vi "drive at angle.vi"() -> ()   [LabVIEW 2016]
uses:
  <vilib>/Rock Robotics/WPI/RobotDrive/WPI_RobotDriveDevRef.ctl
  <vilib>/Rock Robotics/WPI/MotorControl/WPI_MotorControlDeviceRef.ctl
  <vilib>/Rock Robotics/WPI/MotorControl/WPI_MotorControlType.ctl
  <vilib>/Rock Robotics/SystemInterfaces/DIO/FPGA_DIOPWMChannel.ctl
  <vilib>/Rock Robotics/WPI/PWM/WPI_PWMDeadband.ctl
  Robot Global Data.vi
  <vilib>/Rock Robotics/WPI/RobotDrive/WPI_RobotDriveArcadeDrive_Standard(NoSaturation).vi
panel:
  in  "angle":dbl
  in  "power(neg)":dbl
  in  "x inches":dbl
  in  "error in (no error)":errorcluster
  in  "RobotDriveDevRef":T1={"DevStatus"={"status"=FALSE, "code"=0, "source"=""}, "Motors[]"=[], "Square Inputs"=FALSE, "Max Output"=1.0}
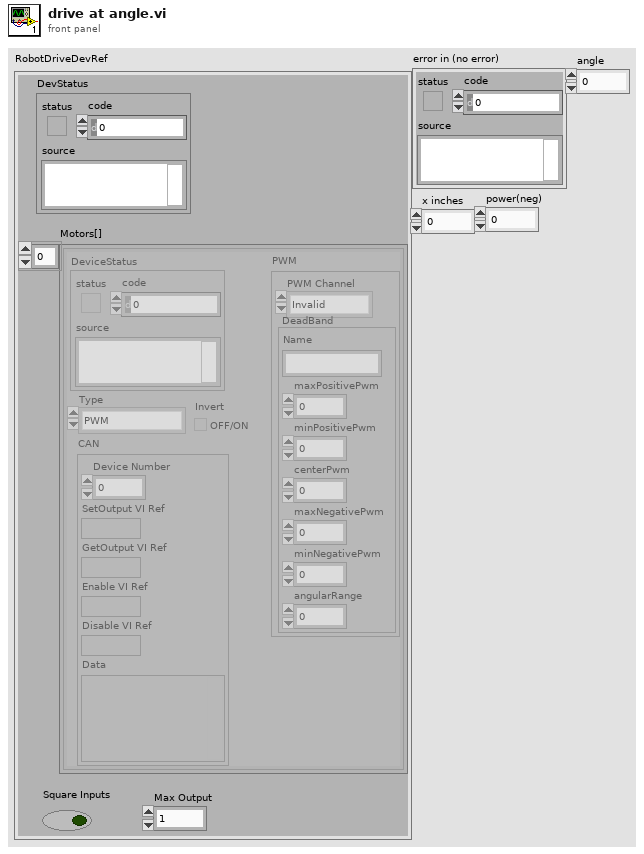
[diagram p1: front panel]
types:
  T1 = typedef "WPI_RobotDriveDevRef.ctl" = cluster{"DevStatus":errorcluster, "Motors[]":T2[], "Square Inputs":bool, "Max Output":dbl}
  T2 = typedef "WPI_MotorControlDeviceRef.ctl" = cluster{"DeviceStatus":errorcluster, "Type":T3, "PWM":cluster{"PWM Channel":T4, "DeadBand":T5}, "CAN":cluster{"Device Number":u8, "SetOutput VI Ref":variant, "GetOutput VI Ref":variant, "Enable VI Ref":variant, "Disable VI Ref":variant, "Data":variant}, "Invert":bool}
  T3 = typedef "WPI_MotorControlType.ctl" = enum16{"PWM", "CAN"}
  T4 = typedef "FPGA_DIOPWMChannel.ctl" = enum8{"PWM 0", "PWM 1", "PWM 2", "PWM 3", "PWM 4", "PWM 5", "PWM 6", "PWM 7", "PWM 8", "PWM 9", "PWM MXP 0", "PWM MXP 1", "PWM MXP 2", "PWM MXP 3", "PWM MXP 4", "PWM MXP 5", "PWM MXP 6", "PWM MXP 7", "PWM MXP 8", "PWM MXP 9", "Invalid"}
  T5 = typedef "WPI_PWMDeadband.ctl" = cluster{"Name":string, "maxPositivePwm":i32, "minPositivePwm":i32, "centerPwm":i32, "maxNegativePwm":i32, "minNegativePwm":i32, "angularRange":u16}
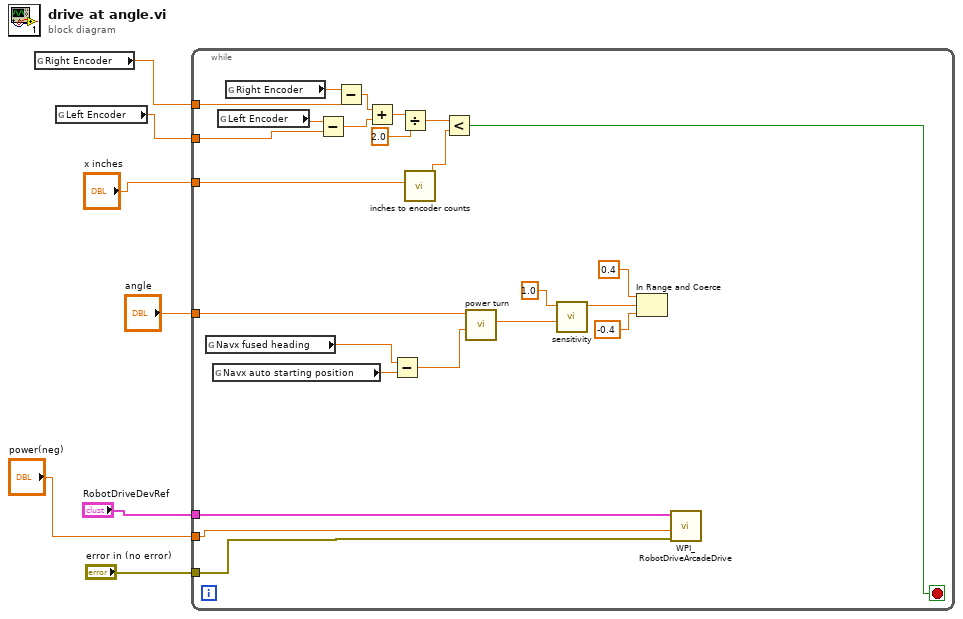
[diagram p0: block diagram]
diagram:
  n1 = global read "Robot Global Data.vi" "Right Encoder"() -> (w7:dbl)
  n2 = global read "Robot Global Data.vi" "Left Encoder"() -> (w6:dbl)
  n3 = while {
    tunnel: w7 -> [w23]
    tunnel: w6 -> [w22]
    tunnel: "RobotDriveDevRef" -> [w21]
    tunnel: "error in (no error)" -> [w20]
    tunnel: "x inches" -> [w19]
    tunnel: "power(neg)" -> [w18]
    tunnel: "angle" -> [w13]
    stop <- w17 stop-if-true
    n4 = global read "Robot Global Data.vi" "Navx fused heading"() -> (w15:dbl)
    n5 = global read "Robot Global Data.vi" "Navx auto starting position"() -> (w16:dbl)
    n6 = global read "Robot Global Data.vi" "Left Encoder"() -> (w30:dbl)
    n7 = global read "Robot Global Data.vi" "Right Encoder"() -> (w31:dbl)
    n8 = Subtract(x=w30, y=w22) -> (x-y=w28:dbl)
    n9 = Subtract(x=w31, y=w23) -> (x-y=w29:dbl)
    n10 = Add(x=w29, y=w28) -> (x+y=w27:dbl)
    n11 = Subtract(x=w15, y=w16) -> (x-y=w14:dbl)
    n12 = Divide(x=w27, y=2.0) -> (x/y=w25:dbl)
    n13 = call "inches to encoder counts.vi"("x inches"=w19) -> ("encoder counts"=w24:dbl)  [unwired: 10 in]
    n14 = Less?(x=w25, y=w24) -> (x < y?=w17:bool)
    n15 = call "power turn.vi"("current angle"=w14, "desired angle(degrees)"=w13) -> ("output"=w12:dbl)  [unwired: 9 in]
    n16 = call "sensitivity.vi"("x"=w12, "sensitivity"=1.0) -> ("scaled value"=w10:dbl)  [unwired: 9 in]
    n17 = In Range and Coerce(upper limit=0.4, x=w10, lower limit=-0.4) -> ()  [unwired: 2 out]
    n18 = call-poly <vilib>:"WPI_RobotDriveArcadeDrive.vi"("error in (no error)"=w20, "Y axis value"=w18, "RobotDriveDevRef"=w21) -> ()  [unwired: 6 in, 3 out]
  }
